vi "LuaVIEW Set Object Attribute.vi"(0 "key":string, 5 "LuaVIEW reference in":T1, 11 "error in (no error)":errorcluster) -> (6 "LuaVIEW reference out":T1, 15 "error out":errorcluster)   [LabVIEW 2013]
doc: "Sets an attribute on a LuaVIEW object. When calling this VI, the value to set (any type) must be at the top of the stack and be preceeded by the object on which to set the attribute. The value being set is removed from the stack. The function's documentation should list these attributes. Note that attributes are read-only on the Lua side. Object attributes can be read from in the very same way as table attributes.\n\nAttributes can be used to adorn an object being returned by a LuaVIEW function with invariant object properties. An alternative use is for an attribute to maintain some object-instance specific variable that changes between method calls, e.g. something like the read/write/seek offset associated with a file handle."
uses:
  typedefs/t_LuaVIEW Reference.ctl
  typedefs/et_LuaVIEW CIN Actions.ctl
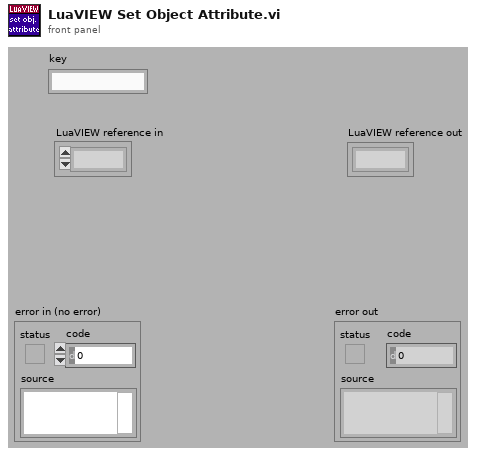
[diagram p1: front panel]
types:
  T1 = typedef "t_LuaVIEW Reference.ctl" = refnum<k1>
  T2 = typedef "et_LuaVIEW CIN Actions.ctl" = enum16{"checksynopsis", "_open", "_registerpublic", "_registerexport", "__never_an_error_result_ns", "luaversion", "cinversion", "_totals", "_taskcount", "pathological", "_unregnextpublic", "registryusecount", "__per_state_actions", "regsetprivate", "regsetindex", "regsetmodule", "_revokeexports", "_usepublic", "prepare", "compile", "execute", "call", "unregstaterefs", "_close", "pullboolean", "pullnumber", "pullI8", "pullU8", "pullI16", "pullU16", "pullI32", "pullU32", "pullobject", "pullrefnum", "pullstring", "pullflat", "pushflat", "pushobject", "getattribute", "setattribute", "stacktostring", "_startyieldtest", "_endyieldtest", "_pollprintbuffer", "__never_an_error_result_ps", "_pollexport", "setclone", "forcecleanup", "gettop", "clearstack", "insert", "pushboolean", "pushnumber", "pushrefnum", "pushstring", "pushnil", "pushvalue", "gettaskref", "settaskref"}
  T3 = typedef "et_LuaVIEW CIN Results.ctl" = enum16{"OK", "error", "main", "call", "clonecall", "modulecall", "exportcall", "index", "yield"}
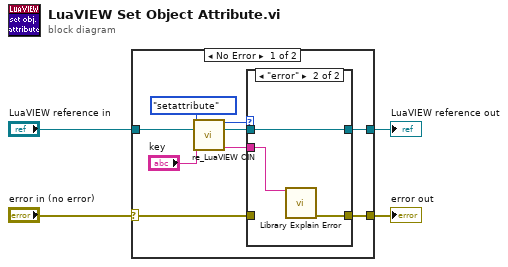
[diagram p0: block diagram]
diagram:
  n1 = case shown="No Error" "error in (no error)" {
    selector: "error in (no error)" -> [w5 w20]
    tunnel: [w8 w19] -> w4
    tunnel: [w6 w20] -> w3
    tunnel: "LuaVIEW reference in" -> [w12 w19]
    frame No Error {
      n2 = call "re_LuaVIEW CIN.vi"("action"=et_LuaVIEW_CIN_Actions."setattribute", "LuaVIEW reference in"=w12, "string in"="key") -> ("result"=w10:T3, "LuaVIEW reference out"=w9:T1, "string out"=w7:string)  [unwired: 6 in, 4 out]
      n3 = case shown="\"error\"" w10 {
        tunnel: [w15 w17] -> w8
        tunnel: w9 -> [w15 w17]
        tunnel: w7 -> [_ w16]
        tunnel: [w14 w18] -> w6
        tunnel: w5 -> [w14 _]
        frame Default {
        }
        frame "error" {
          n4 = call "Library Explain Error.vi"("explanation prefix (none)"=w16) -> ("explained error"=w18:errorcluster)  [unwired: 14 in]
        }
      }
    }
    frame Error {
    }
  }
  "LuaVIEW reference out" <- w4
  "error out" <- w3
